vi "PH_GUI.set shutter GUI object.vi"(1 "Wanted Boolean Ref":refnum<vi>, 2 "Tip Strip":string="N/A", 3 "Shutter State":T1, 4 "Disabled? (false)":bool, 5 "error in (no error)":errorcluster) -> (19 "error out":errorcluster)   [LabVIEW 2014, in "PH_Common.lvlib"]
doc: "This VI sets two boolean Controls (\"Ref In\" and \"Ref Out\") depending on the \"Shutter State\":\n\nNo Link and Default:\nboth visible, both blinking, both disabled, and both colors = blue\n\nNo Info:\nboth visible, both not blinking, both disabled, and both colors = blue\n\nIn: \nIn visible, Out not visible, both not blinking, both \"Disabled\", and both colors = lightgreen\n\nOut:\nOut visible, In not visible, both not blinking, both \"Disabled\", and both colors = lightgreen\n\nin between:\nboth visible, both not blinking, both \"Disabled\", and both colors = yellow"
uses:
  PH_Common.lvlib
  PHELIX/PH_BL-Master/PH_BL-Master.Shutter State.ctl
  PHELIX/PH_BL-Master/PH_BL-Master.lvlib
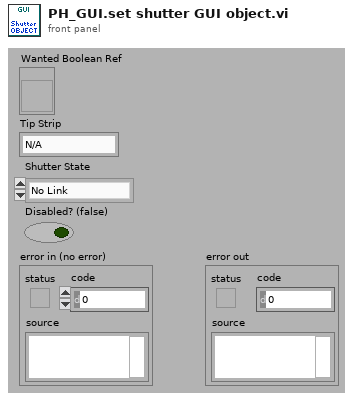
[diagram p1: front panel]
types:
  T1 = typedef "PH_BL-Master.lvlib/PH_BL-Master.Shutter State.ctl" = enum16{"No Link", "No Info", "In", "Out", "in between"}
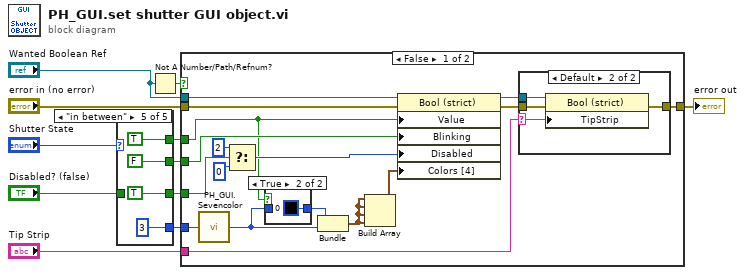
[diagram p0: block diagram]
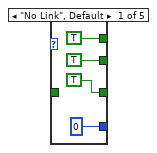
[diagram p5: hidden frame]
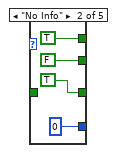
[diagram p6: hidden frame]
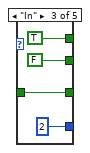
[diagram p7: hidden frame]
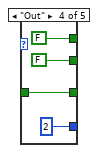
[diagram p8: hidden frame]
diagram:
  n1 = case shown="\"in between\"" "Shutter State" {
    tunnel: [TRUE FALSE FALSE FALSE FALSE] -> w4
    tunnel: [TRUE TRUE w21 w25 TRUE] -> w3
    tunnel: [0 ("State") 0 ("State") 2 ("State") 2 ("State") 3 ("State")] -> w8
    tunnel: "Disabled? (false)" -> [_ _ w21 w25 _]
    tunnel: [TRUE TRUE TRUE FALSE TRUE] -> w2
    frame "No Link", Default {
    }
    frame "No Info" {
    }
    frame "In" {
    }
    frame "Out" {
    }
    frame "in between" {
    }
  }
  n2 = Not A Number/Path/Refnum?(number/path/refnum="Wanted Boolean Ref") -> (NaN/Path/Refnum?=w6:bool)
  n3 = case shown="False" w6 {
    tunnel: "Wanted Boolean Ref" -> [w48 _]
    tunnel: "error in (no error)" -> [w47 w56]
    tunnel: [w34 w56] -> w10
    tunnel: w4 -> [w46 _]
    tunnel: w3 -> [w42 _]
    tunnel: w8 -> [w41 _]
    tunnel: w2 -> [w37 _]
    tunnel: "Tip Strip" -> [w32 _]
    frame False {
      n4 = call "PH_GUI.Sevencolor.vi"("State"=w41) -> ("Color Box"=w36:u32)
      n5 = Select(t=u8 2 ("Disabled"), s=w42, f=u8 0 ("Disabled")) -> (s? t:f=w43:u8)
      n6 = case shown="True" w37 {
        tunnel: [w54 u32 0 ("Color Box")] -> w38
        tunnel: w36 -> [w54 _]
        frame False {
        }
        frame True {
        }
      }
      n7 = Bundle("Color Box"=w38, "Color Box"=w36) -> (w40:cluster{"Color Box":u32, "Color Box":u32})  [unwired: 1 in]
      n8 = Build Array(w40, w40, w40, w40) -> (w39:cluster{"Color Box":u32, "Color Box":u32}[])
      n9 = property class="Bool (strict)"(reference=w48, error in=w47, "Value"=w37, "Blinking"=w46, "Disabled"=w43, "Colors [4]"=w39) -> (reference out=w33:refnum<vi>, error out=w35:errorcluster)
      n10 = case shown="Default" w32 {
        selector: w32 -> [_ w50]
        tunnel: w35 -> [w49 w53]
        tunnel: [w49 w52] -> w34
        tunnel: w33 -> [_ w51]
        frame "", "N/A" {
        }
        frame Default {
          n11 = property class="Bool (strict)"(reference=w51, error in=w53, "TipStrip"=w50) -> (error out=w52:errorcluster)  [unwired: 1 out]
        }
      }
    }
    frame True {
    }
  }
  "error out" <- w10
